vi "CarWashTestcase.vi"(11 "error in":errorcluster) -> (15 "error out":errorcluster)   [LabVIEW 2016]
uses:
  <vilib>/addons/_JKI Toolkits/Caraya/classes/Test/Test.lvclass
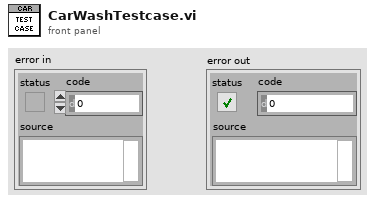
[diagram p1: front panel]
types:
  T1 = typedef "Wash Step Config.ctl" = cluster{"Wash Option":string, "Car Position":i32, "Elapsed Time":dbl}
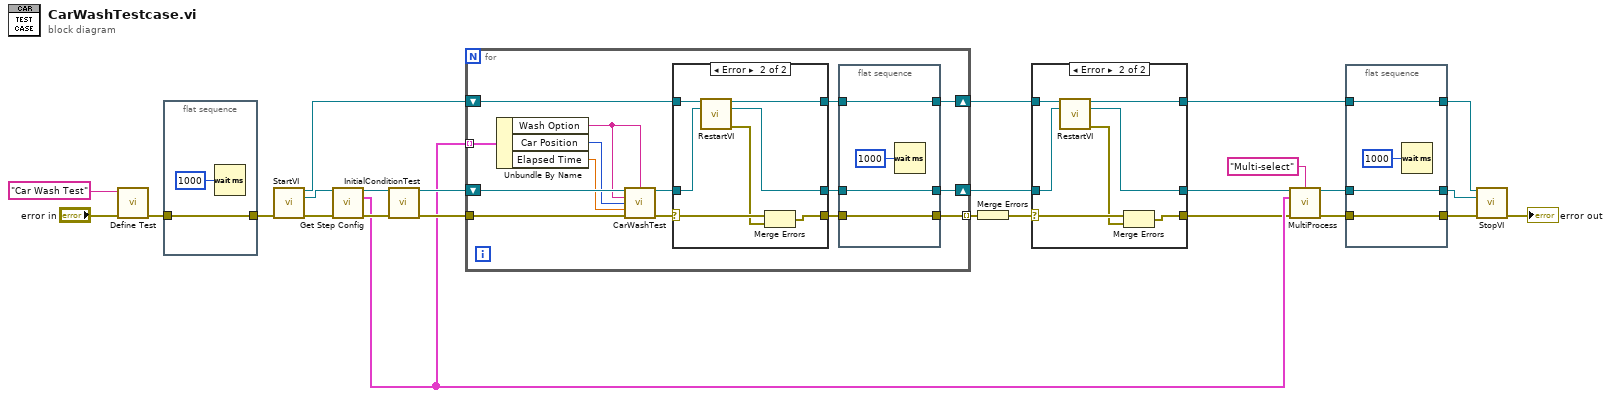
[diagram p0: block diagram]
diagram:
  n1 = call <vilib>:"Define Test.vi"("error in (no error)"="error in", "Label (VI Title)"="Car Wash Test" ("Label")) -> ("error out"=w8:errorcluster)  [unwired: 9 in]
  n2 = flat-sequence {
    tunnel: [w27] -> w7
    tunnel: w8 -> [w27]
    frame #0 {
      n3 = Wait (ms)(milliseconds to wait=u32 1000) -> ()  [unwired: 1 out]
    }
  }
  n4 = call "StartVI.vi"("error in"=w7) -> ("Application Ref out"=w21:refnum<vi>, "VI Reference"=w18:refnum<vi>, "error out"=w16:errorcluster)  [unwired: 12 in]
  n5 = call "Get Step Config.vi"("VI In"=w18, "error in"=w16) -> ("VI out"=w17:refnum<vi>, "Wash Array"=w14:T1[], "error out"=w15:errorcluster)  [unwired: 11 in]
  n6 = call "InitialConditionTest.vi"("VI Reference In"=w17, "error in"=w15) -> ("VI Reference Out"=w25:refnum<vi>, "error out"=w26:errorcluster)  [unwired: 12 in]
  n7 = for {
    shift-right: [w31] -> w5
    shift-left: w25 -> [w42]
    tunnel: w14 -> [w41] mode=indexing
    tunnel: w26 -> [w43]
    tunnel: [w34] -> w19 mode=indexing
    shift-right: [w30] -> w6
    shift-left: w21 -> [w35]
    n8 = Unbundle By Name(w41) -> ("Wash Option"=w38:string, "Car Position"=w40:i32, "Elapsed Time"=w39:dbl)
    n9 = call "CarWashTest.vi"("VI Reference In"=w42, "Label"=w38, "Wash Option"=w38, "Car Position"=w40, "Elapsed Time"=w39, "error in"=w43) -> ("VI Reference Out"=w36:refnum<vi>, "error out"=w37:errorcluster)  [unwired: 8 in]
    n10 = case shown="Error" w37 {
      selector: w37 -> [w49 w57]
      tunnel: [w49 w56] -> w33
      tunnel: w36 -> [w50 w53]
      tunnel: [w50 w54] -> w32
      tunnel: [w48 w51] -> w29
      tunnel: w35 -> [w48 w52]
      frame No Error {
      }
      frame Error {
        n11 = call "RestartVI.vi"("Application Ref in"=w52, "VI in"=w53) -> ("Application Ref out"=w51:refnum<vi>, "VI out"=w54:refnum<vi>, "error out"=w55:errorcluster)  [unwired: 11 in]
        n12 = Merge Errors(w57, w55) -> (w56:errorcluster)
      }
    }
    n13 = flat-sequence {
      tunnel: [w47] -> w34
      tunnel: w33 -> [w47]
      tunnel: w32 -> [w46]
      tunnel: [w46] -> w31
      tunnel: [w45] -> w30
      tunnel: w29 -> [w45]
      frame #0 {
        n14 = Wait (ms)(milliseconds to wait=u32 1000) -> ()  [unwired: 1 out]
      }
    }
  }
  n15 = Merge Errors(w19) -> (w2:errorcluster)
  n16 = case shown="Error" w2 {
    selector: w2 -> [w59 w67]
    tunnel: [w59 w66] -> w1
    tunnel: w5 -> [w60 w63]
    tunnel: [w60 w64] -> w4
    tunnel: [w58 w61] -> w3
    tunnel: w6 -> [w58 w62]
    frame No Error {
    }
    frame Error {
      n17 = call "RestartVI.vi"("Application Ref in"=w62, "VI in"=w63) -> ("Application Ref out"=w61:refnum<vi>, "VI out"=w64:refnum<vi>, "error out"=w65:errorcluster)  [unwired: 11 in]
      n18 = Merge Errors(w67, w65) -> (w66:errorcluster)
    }
  }
  n19 = call "MultiProcess.vi"("VI Reference In"=w4, "Label"="Multi-select", "Wash Array"=w14, "error in"=w1) -> ("VI Reference Out"=w13:refnum<vi>, "error out"=w11:errorcluster)  [unwired: 10 in]
  n20 = flat-sequence {
    tunnel: [w71] -> w9
    tunnel: w11 -> [w71]
    tunnel: w13 -> [w68]
    tunnel: [w70] -> w10
    tunnel: w3 -> [w70]
    tunnel: [w68] -> w12
    frame #0 {
      n21 = Wait (ms)(milliseconds to wait=u32 1000) -> ()  [unwired: 1 out]
    }
  }
  n22 = call "StopVI.vi"("Application Ref in"=w10, "VI in"=w12, "error in (no error)"=w9) -> ("error out"=→"error out":errorcluster)  [unwired: 12 in]
